vi "NT Publish Match Info.vi"(8 "error in (no error)":errorcluster, 11 "NT Variable Name":string) -> (0 "error out":errorcluster, 3 "Match Info String":string)   [LabVIEW 2018]
uses:
  <vilib>/Rock Robotics/Network Tables/NT Write String.vi
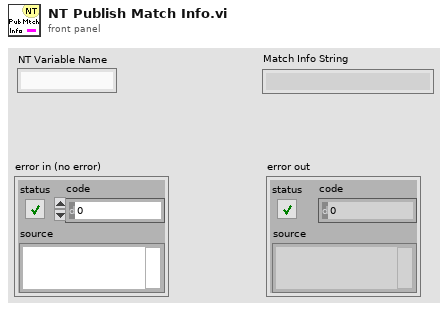
[diagram p1: front panel]
types:
  T1 = typedef "NetComm_MatchType.ctl" = enum32{"None", "Practice", "Qualification", "Elimination"}
  T2 = typedef "WPI_DriverStationPositionInfo.ctl" = enum16{"1", "2", "3"}
  T3 = typedef "WPI_DriverStationAllianceInfo.ctl" = enum16{"Red", "Blue", "Invalid"}
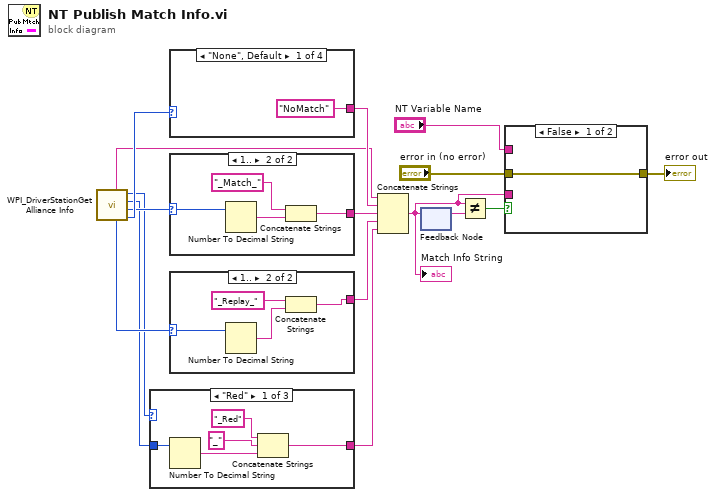
[diagram p0: block diagram]
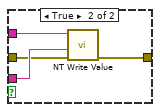
[diagram p2: hidden frame]
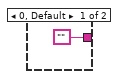
[diagram p3: hidden frame]
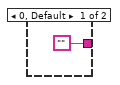
[diagram p4: hidden frame]
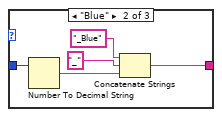
[diagram p5: hidden frame]
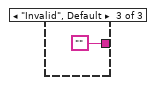
[diagram p6: hidden frame]
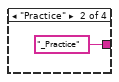
[diagram p7: hidden frame]
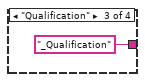
[diagram p8: hidden frame]
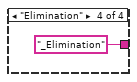
[diagram p9: hidden frame]
diagram:
  n1 = call <vilib>:"WPI_DriverStationGet Alliance Info.vi"() -> ("Match Type"=w15:T1, "Match Number"=w7:u16, "Position"=w6:T2, "Alliance"=w5:T3, "Replay Number"=w9:u16, "Event Name"=w4:string)  [unwired: 6 in]
  n2 = case shown="\"Red\"" w5 {
    tunnel: [w18 w22 ""] -> w12
    tunnel: w6 -> [w17 w26 _]
    frame "Red" {
      n3 = Number To Decimal String(number=w17) -> (decimal integer string=w19:string)  [unwired: 1 in]
      n4 = Concatenate Strings("_Red", "_", w19) -> (w18:string)
    }
    frame "Blue" {
      n5 = Number To Decimal String(number=w26) -> (decimal integer string=w23:string)  [unwired: 1 in]
      n6 = Concatenate Strings("_Blue", "_", w23) -> (w22:string)
    }
    frame "Invalid", Default {
    }
  }
  n7 = case shown="\"None\", Default" w15 {
    tunnel: ["NoMatch" "_Practice" "_Qualification" "_Elimination"] -> w11
    frame "None", Default {
    }
    frame "Practice" {
    }
    frame "Qualification" {
    }
    frame "Elimination" {
    }
  }
  n8 = case shown="1.." w7 {
    selector: w7 -> [_ w33]
    tunnel: ["" w34] -> w8
    frame 0, Default {
    }
    frame 1.. {
      n9 = Number To Decimal String(number=w33) -> (decimal integer string=w35:string)  [unwired: 1 in]
      n10 = Concatenate Strings("_Match_", w35) -> (w34:string)
    }
  }
  n11 = case shown="1.." w9 {
    selector: w9 -> [_ w41]
    tunnel: ["" w38] -> w10
    frame 0, Default {
    }
    frame 1.. {
      n12 = Number To Decimal String(number=w41) -> (decimal integer string=w39:string)  [unwired: 1 in]
      n13 = Concatenate Strings("_Replay_", w39) -> (w38:string)
    }
  }
  n14 = Concatenate Strings(w4, w11, w8, w10, w12) -> (w1:string)
  "Match Info String" <- w1
  n15 = feedback #1() -> (w13:string)  [unwired: 1 in]
  n16 = feedback-in #1(w1) -> ()
  n17 = Not Equal?(x=w1, y=w13) -> (x != y?=w14:bool)
  n18 = case shown="False" w14 {
    tunnel: w1 -> [_ w46]
    tunnel: "NT Variable Name" -> [_ w45]
    tunnel: "error in (no error)" -> [w42 w44]
    tunnel: [w42 w43] -> w2
    frame False {
    }
    frame True {
      n19 = call-poly <vilib>:"NT Write Value.vi"("error in"=w44, "String"=w46, "Name"=w45) -> ("error out"=w43:errorcluster)  [unwired: 8 in]
    }
  }
  "error out" <- w2
